vi "Enable Item.vi"(8 "error in (no error)":errorcluster, 10 "Item Name":string, 11 "Module Name":string) -> (0 "error out":errorcluster)   [LabVIEW 2020, in "Group Interface.lvlib"]
uses:
  Group Interface.lvlib
  <userlib>/_NEVSTOP/Communicable State Machine(CSM)/Communicable State Machine.lvlib
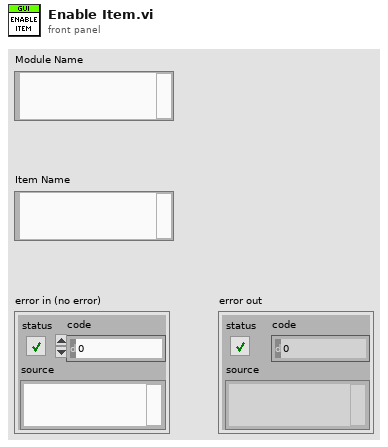
[diagram p1: front panel]
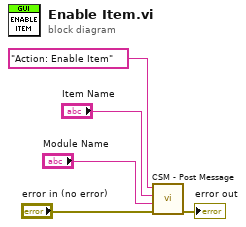
[diagram p0: block diagram]
diagram:
  n1 = call <userlib>:"CSM - Post Message.vi"("Error In (No Error)"="error in (no error)", "Target Module"="Module Name", "Arguments (\"\")"="Item Name", "State"="Action: Enable Item") -> ("error out"=→"error out":errorcluster)  [unwired: 7 in]
